vi "ReadMark10Events.vi"(8 "Error In":errorcluster) -> (0 "Error Out":errorcluster, 3 "EventLog":string)   [LabVIEW 2019, in "Mark 10 TSTM-DC.lvlib" / "Mark 10 Event Monitor.lvlib"]
uses:
  Mark 10 Event Monitor.lvlib
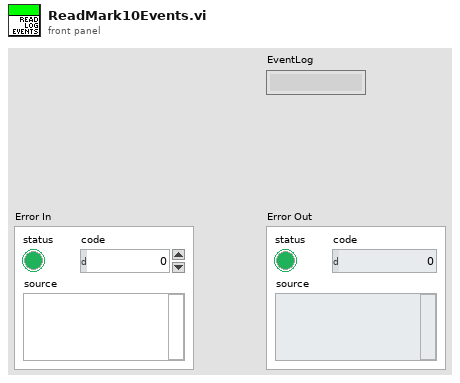
[diagram p1: front panel]
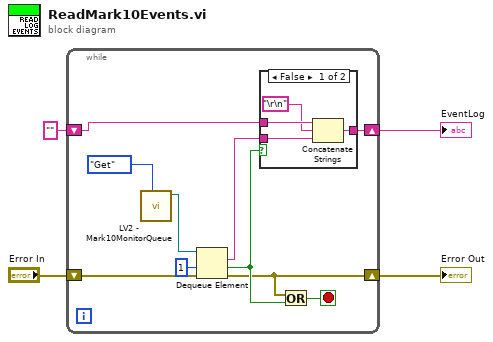
[diagram p0: block diagram]
diagram:
  n1 = while {
    shift-right: [w5] -> w3
    shift-left: "Error In" -> [w14]
    shift-right: [w9] -> w2
    shift-left: "" ("String") -> [w8]
    stop <- w6 stop-if-true
    n2 = call "LV2 - Mark10MonitorQueue.vi"("Enum"=enum16{"Set", "Get"}."Get") -> ("Mark10Monitor out"=w12:refnum<queue>)  [unwired: 10 in]
    n3 = Dequeue Element(queue=w12, timeout in ms (-1)=1, error in (no error)=w14) -> (element=w11:string, timed out?=w7:bool, error out=w5:errorcluster)  [unwired: 1 out]
    n4 = case shown="False" w7 {
      tunnel: w11 -> [w18 _]
      tunnel: [w17 w19] -> w9
      tunnel: w8 -> [w16 w19]
      frame False {
        n5 = Concatenate Strings(w16, "\r\n", w18) -> (w17:string)
      }
      frame True {
      }
    }
    n6 = Or(x=w5, y=w7) -> (x .or. y?=w6:bool)
  }
  "Error Out" <- w3
  "EventLog" <- w2
